vi "Charge.vi"(8 "error in (no error)":errorcluster, 11 "GumballMachine in":refnum<class "GumballMachine.lvclass">) -> (0 "error out":errorcluster, 2 "ProcessMessage":string, 3 "GumballMachine out":refnum<class "GumballMachine.lvclass">)   [LabVIEW 2013, in "GumballMachine.lvclass"]
uses:
  GumballMachine.lvclass
  GumballMachine.lvclass/GumballMachine.ctl
  State.lvclass/State.lvclass
  StateMark.ctl
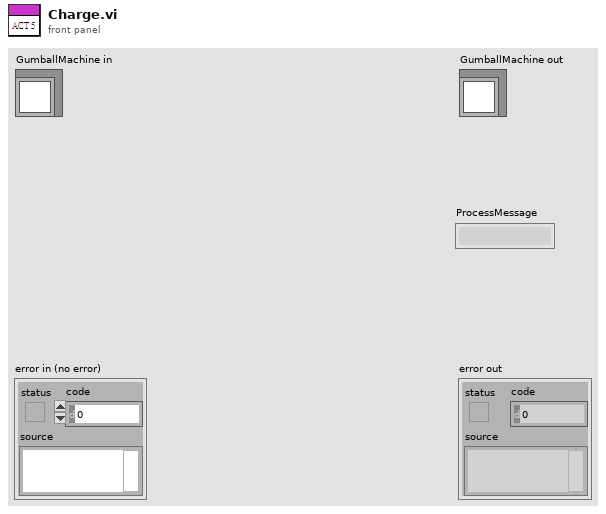
[diagram p1: front panel]
types:
  T1 = typedef "StateMark.ctl" = enum16{"沒有硬幣", "有硬幣", "賣出糖果", "糖果賣完", "NoChange"}
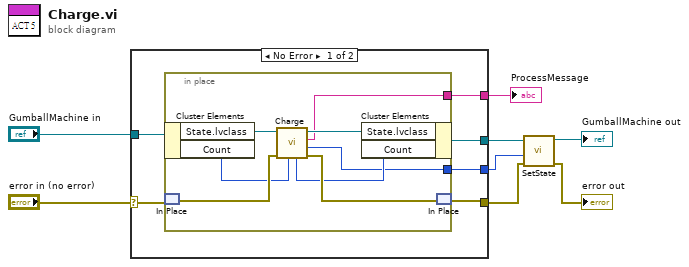
[diagram p0: block diagram]
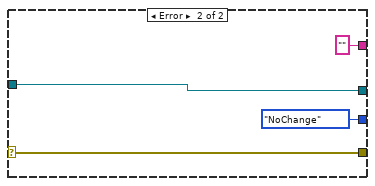
[diagram p2: hidden frame]
diagram:
  n1 = case shown="No Error" "error in (no error)" {
    selector: "error in (no error)" -> [w14 w26]
    tunnel: [w12 w26] -> w3
    tunnel: [w11 w25] -> w5
    tunnel: "GumballMachine in" -> [w13 w25]
    tunnel: [w10 "" ("ProcessMessage")] -> w6
    tunnel: [w9 StateMark."NoChange" ("NextState")] -> w2
    frame No Error {
      n2 = in-place {
        in-place-border: [w18] -> w10
        in-place-border: [w15] -> w9
        n3 = in-place-cluster #1(w13) -> ("State.lvclass"=w22:refnum<class "State.lvclass">, "Count"=w17:i32)
        n4 = in-place-match #2(w14) -> (w20:errorcluster)
        n5 = call-dynamic "Charge.vi"("Count"=w17, "error in (no error)"=w20, "State in"=w22) -> ("error out"=w19:errorcluster, "NextState"=w15:T1, "ProcessMessage"=w18:string, "State out"=w21:refnum<class "State.lvclass">, "Count Out"=w16:i32)  [unwired: 4 in]
        n6 = in-place-cluster #1("State.lvclass"=w21, "Count"=w16) -> (w11:refnum<class "GumballMachine.lvclass">)
        n7 = in-place-match #2(w19) -> (w12:errorcluster)
      }
    }
    frame Error {
    }
  }
  "ProcessMessage" <- w6
  n8 = call-dynamic "SetState.vi"("error in (no error)"=w3, "State"=w2, "GumballMachine in"=w5) -> ("error out"=→"error out":errorcluster, "GumballMachine out"=→"GumballMachine out":refnum<class "GumballMachine.lvclass">)  [unwired: 7 in]
